vi "Create Queue.vi"(8 "error in (no error)":errorcluster) -> (0 "error out":errorcluster, 3 "Queue out":refnum<queue>)   [LabVIEW 2016]
uses:
  Controls/Message Structure.ctl
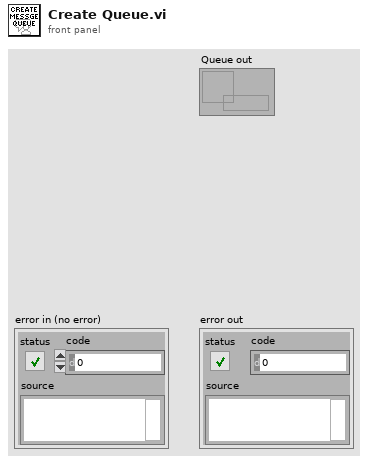
[diagram p1: front panel]
types:
  T1 = typedef "Message Structure.ctl" = cluster{"Data":variant, "Cmd":string}
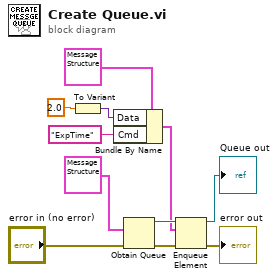
[diagram p0: block diagram]
diagram:
  n1 = To Variant(anything=2.0) -> (Variant=w3:variant)
  n2 = Bundle By Name(cluster=T1 {"Data"=variant, "Cmd"=""} ("Message"), "Data"=w3, "Cmd"="ExpTime") -> (w1:T1)
  n3 = Obtain Queue(element data type=T1 {"Data"=variant, "Cmd"=""}, error in (no error)="error in (no error)") -> (queue out=w8:refnum<queue>, error out=w9:errorcluster)  [unwired: 3 in, 1 out]
  n4 = Enqueue Element(queue=w8, element=w1, error in (no error)=w9) -> (queue out=→"Queue out":refnum<queue>, error out=→"error out":errorcluster)  [unwired: 1 in, 1 out]
